vi "Process PA Compass Data.vi"(11 "RDS State in":refnum<class "RDS State.lvclass">) -> (3 "RDS State out":refnum<class "RDS State.lvclass">)   [LabVIEW 2015]
uses:
  RDS State.lvclass
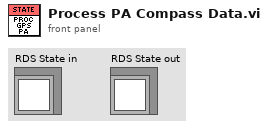
[diagram p1: front panel]
types:
  T1 = typedef "RDS Instrument Library.lvlib/Compass Data.ctl" = cluster{"Compass Heading":dbl, "pitch Angle":dbl, "roll Angle":dbl, "Temperature":dbl, "Depth":dbl, "Magnetic Field":dbl, "Magnetic Field X":dbl, "Magnetic Field Y":dbl, "Magnetic Field Z":dbl, "Acceleration":dbl, "Acceleration X":dbl, "Acceleration Y":dbl, "Gyro":dbl, "Gyro X":dbl, "Acceleration Z":dbl, "Gyro Y":dbl}
  T2 = typedef "Processed PA Block.ctl" = cluster{"GPS Heading":dbl, "GPS Speed":dbl, "GPS Latitude":ext, "GPS Longitude":ext, "Compass heading":dbl, "Pitch":dbl, "Roll":dbl}
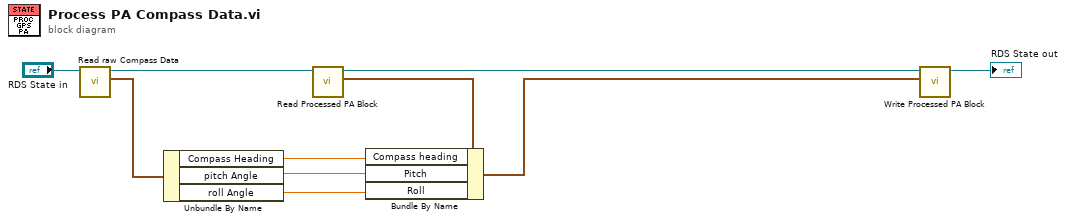
[diagram p0: block diagram]
diagram:
  n1 = call "Read raw Compass Data.vi"("RDS State in"="RDS State in") -> ("Compass Data"=w5:T1, "RDS State out"=w7:refnum<class "RDS State.lvclass">)  [unwired: 8 in, 1 out]
  n2 = Unbundle By Name(w5) -> ("Compass Heading"=w4:dbl, "pitch Angle"=w3:dbl, "roll Angle"=w2:dbl)
  n3 = call "Read Processed PA Block.vi"("RDS State in"=w7) -> ("Processed PA Block"=w8:T2, "RDS State out"=w9:refnum<class "RDS State.lvclass">)  [unwired: 8 in, 1 out]
  n4 = Bundle By Name(cluster=w8, "Compass heading"=w4, "Pitch"=w3, "Roll"=w2) -> (w1:T2)
  n5 = call "Write Processed PA Block.vi"("Processed PA Block"=w1, "RDS State in"=w9) -> ("RDS State out"=→"RDS State out":refnum<class "RDS State.lvclass">)  [unwired: 8 in, 1 out]
